vi "q1 distance.vi"() -> ()   [LabVIEW 2025]
panel:
  out "distance":dbl
  out "(x1-x2)^2":dbl
  in  "y2":dbl
  in  "y1":dbl
  in  "x2":dbl
  in  "x1":dbl
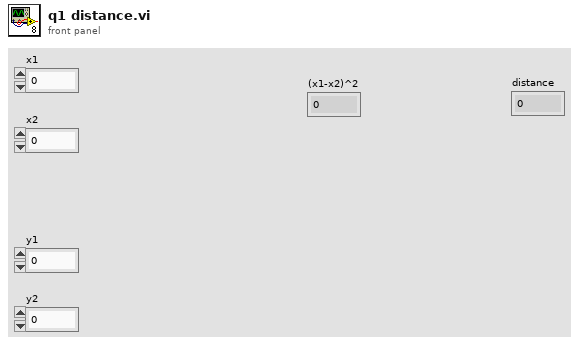
[diagram p1: front panel]
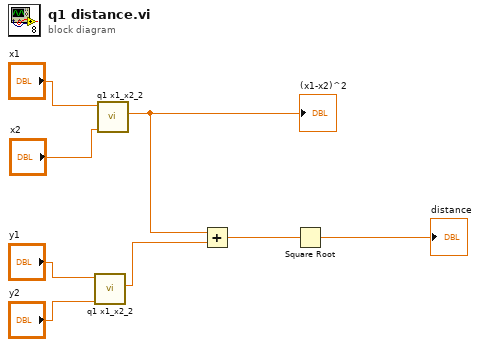
[diagram p0: block diagram]
diagram:
  n1 = call "q1 x1_x2_2.vi"("x2"="y2", "x1"="y1") -> ("(x1-x2)^2"=w3:dbl)  [unwired: 9 in]
  n2 = call "q1 x1_x2_2.vi"("x2"="x2", "x1"="x1") -> ("(x1-x2)^2"=w4:dbl)  [unwired: 9 in]
  "(x1-x2)^2" <- w4
  n3 = Add(x=w4, y=w3) -> (x+y=w2:dbl)
  n4 = Square Root(x=w2) -> (sqrt(x)=→"distance":dbl)
